vi "Add Service VI.vi"(8 "error in (no error)":errorcluster, 9 "RESTful VI configuration":T1={"Service VI Type"=enum."Web Method", "Load VI at statup"=TRUE, "Keep VI in memory"=TRUE, "Output type"=enum."Terminal", "Output format"=enum."XML", "Use headers"=TRUE, "Buffered"=TRUE, "eng_Load VI by name"=FALSE}, 10 "ProjectItem Refnum":refnum<vi>, 11 "NI_AB_API_RESTful in":refnum<class "NI_AB_API_RESTful.lvclass">) -> (0 "error out":errorcluster, 3 "NI_AB_API_RESTful out":refnum<class "NI_AB_API_RESTful.lvclass">)   [LabVIEW 2020, in "NI_AB_API_RESTful.lvclass"]
uses:
  <vilib>/AppBuilder/AB_API/RESTful/NI_AB_API_RESTful.lvclass
  <vilib>/AppBuilder/AB_API/RESTful/NI_AB_API_RESTful.lvclass/NI_AB_API_RESTful.ctl
  <vilib>/AppBuilder/AB_Classes/Source/RESTfulVI/Configure_RESTfulVI/AB_RESTful_VIType.ctl
  <vilib>/AppBuilder/AB_Classes/Source/RESTfulVI/Configure_RESTfulVI/AB_RESTful_OutputType.ctl
  <vilib>/AppBuilder/AB_Classes/Source/RESTfulVI/Configure_RESTfulVI/AB_RESTful_OutputFormat.ctl
  <vilib>/AppBuilder/AB_Classes/Source/RESTfulVI/Configure_RESTfulVI/AB_RESTful_Configuration.ctl
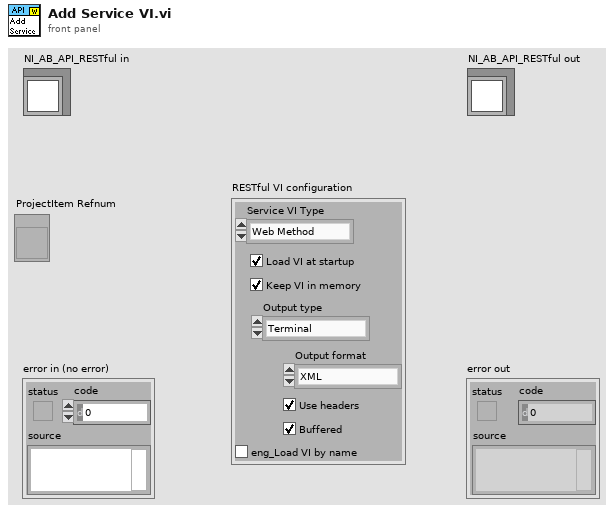
[diagram p1: front panel]
types:
  T1 = typedef "AB_RESTful_Configuration.ctl" = cluster{"Service VI Type":T2, "Load VI at statup":bool, "Keep VI in memory":bool, "Output type":T3, "Output format":T4, "Use headers":bool, "Buffered":bool, "eng_Load VI by name":bool}
  T2 = typedef "AB_RESTful_VIType.ctl" = enum32{"Web Method", "Auxiliary", "eng_Internal", "eng_Content"}
  T3 = typedef "AB_RESTful_OutputType.ctl" = enum32{"Terminal", "Stream"}
  T4 = typedef "AB_RESTful_OutputFormat.ctl" = enum32{"XML", "Text", "HTML", "JSON"}
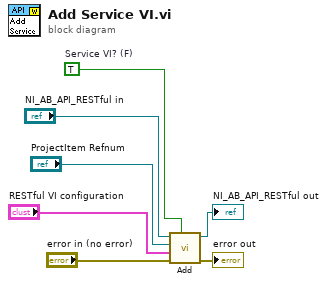
[diagram p0: block diagram]
diagram:
  w7 = TRUE  # Service VI? (F)
  n1 = call <vilib>:"Add.vi"("Service VI? (F)"=w7, "error in (no error)"="error in (no error)", "RESTful VI configuration"="RESTful VI configuration", "ProjectItem Refnum"="ProjectItem Refnum", "NI_AB_API_RESTful in"="NI_AB_API_RESTful in") -> ("error out"=→"error out":errorcluster, "NI_AB_API_RESTful out"=→"NI_AB_API_RESTful out":refnum<class "NI_AB_API_RESTful.lvclass">)  [unwired: 5 in]
